vi "Set Current.vi"(7 "Chanel":string, 10 "Set Current":string, 11 "VISA Source":string) -> (4 "error out":errorcluster)   [LabVIEW 2020]
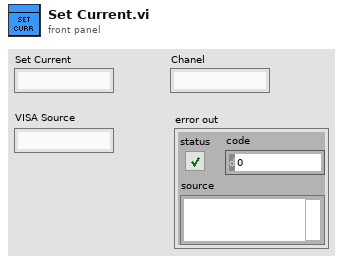
[diagram p1: front panel]
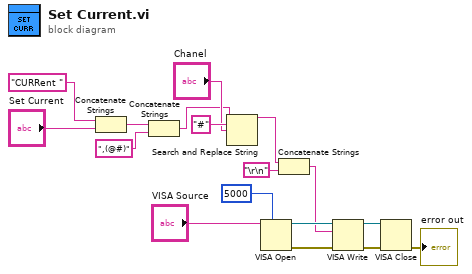
[diagram p0: block diagram]
diagram:
  n1 = Concatenate Strings("CURRent " ("string"), "Set Current") -> (w8:string)
  n2 = Concatenate Strings(w8, ",(@#)" ("string")) -> (w4:string)
  n3 = Search and Replace String(input string=w4, search string="#", replace string="Chanel") -> (result string=w3:string)  [unwired: 5 in, 3 out]
  n4 = VISA Open(timeout (0)=u32 5000 ("VISA Open timeout (0)"), VISA resource name="VISA Source") -> (VISA resource name=w17:refnum<visa-resource-name>, error out=w16:errorcluster)  [unwired: 3 in]
  n5 = Concatenate Strings(w3, "\r\n") -> (w11:string)
  n6 = VISA Write(VISA resource name=w17, write buffer=w11, error in (no error)=w16) -> (VISA resource name out=w14:refnum<visa-resource-name>, error out=w13:errorcluster)  [unwired: 1 out]
  n7 = VISA Close(VISA resource name=w14, error in (no error)=w13) -> (error out=→"error out":errorcluster)
